vi "RestartVI.vi"(0 "Application Ref in":refnum<vi>, 5 "VI in":refnum<vi>, 11 "error in (no error)":errorcluster) -> (4 "Application Ref out":refnum<vi>, 6 "VI out":refnum<vi>, 15 "error out":errorcluster)   [LabVIEW 2016]
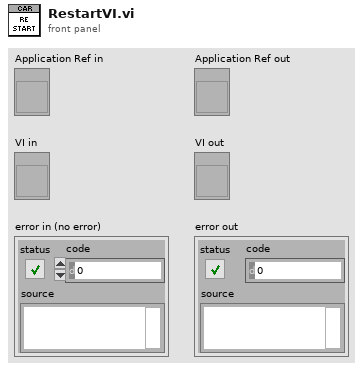
[diagram p1: front panel]
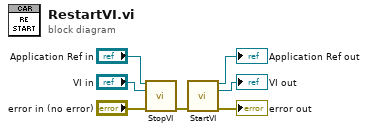
[diagram p0: block diagram]
diagram:
  n1 = call "StopVI.vi"("Application Ref in"="Application Ref in", "VI in"="VI in", "error in (no error)"="error in (no error)") -> ("error out"=w2:errorcluster)  [unwired: 12 in]
  n2 = call "StartVI.vi"("error in"=w2) -> ("Application Ref out"=→"Application Ref out":refnum<vi>, "VI Reference"=→"VI out":refnum<vi>, "error out"=→"error out":errorcluster)  [unwired: 12 in]
